vi "Get Case Structure (by Name).vi"(8 "error in (no error)":errorcluster, 10 "Case Structure name":string, 11 "VI ref in":refnum<vi>) -> (0 "error out":errorcluster, 1 "Found ?":bool, 2 "CaseStructure out":refnum<vi>, 3 "VI ref out":refnum<vi>)   [LabVIEW 2019, in "gRPC Template Creation Utility.lvlib"]
uses:
  gRPC Template Creation Utility.lvlib
  <vilib>/Utility/traverseref.llb/TRef TravTarget.ctl
  <vilib>/Utility/traverseref.llb/VI Scripting - Traverse.lvlib
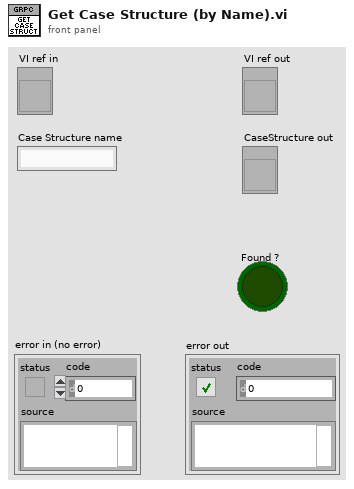
[diagram p1: front panel]
types:
  T1 = typedef "TRef TravTarget.ctl" = enum16{"FP", "BD", "Other"}
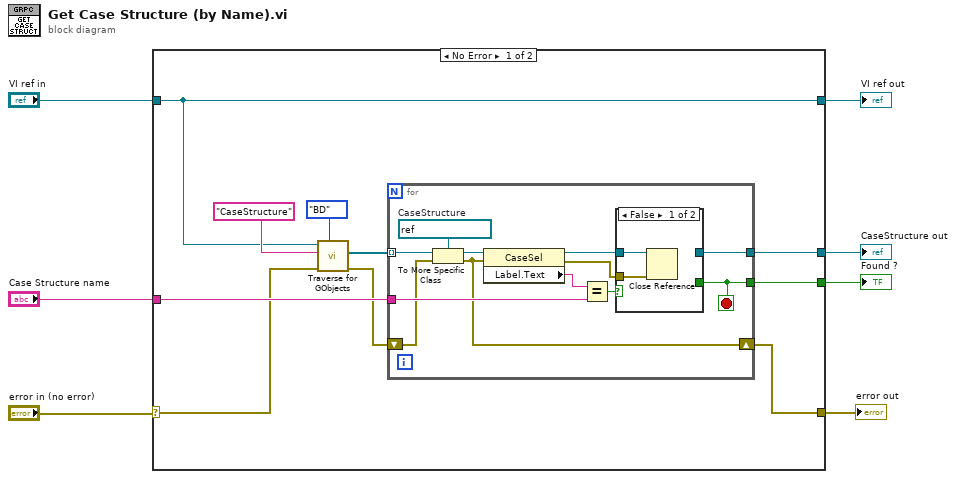
[diagram p0: block diagram]
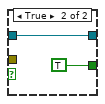
[diagram p2: hidden frame]
diagram:
  n1 = case shown="No Error" "error in (no error)" {
    selector: "error in (no error)" -> [w11 w35]
    tunnel: [w17 _] -> w7
    tunnel: "Case Structure name" -> [w16 _]
    tunnel: "VI ref in" -> [w8 w34]
    tunnel: [w12 _] -> w4
    tunnel: [w9 w35] -> w2
    tunnel: [w8 w34] -> w1
    frame No Error {
      n2 = call <vilib>:"Traverse for GObjects.vi"("Traverse Target"=TRef_TravTarget."BD", "error in (no error)"=w11, "Class Name"="CaseStructure", "VI Refnum"=w8) -> ("error out"=w10:errorcluster, "References"=w15:refnum<vi>[])  [unwired: 4 in, 2 out]
      n3 = for {
        tunnel: w15 -> [w27] mode=indexing
        tunnel: w16 -> [w25]
        tunnel: [w22] -> w17
        tunnel: [w18] -> w12
        shift-right: [w19] -> w9
        shift-left: w10 -> [w21]
        stop <- w18 stop-if-true
        w29 = refnum<vi> refnum  # CaseStructure
        n4 = To More Specific Class(target class=w29, reference=w27, error in=w21) -> (specific class reference=w28:refnum<vi>, error out=w19:errorcluster)
        n5 = property class="CaseSel"(reference=w28, error in=w19) -> (reference out=w23:refnum<vi>, error out=w20:errorcluster, "Label.Text"=w26:string)
        n6 = Equal?(x=w26, y=w25) -> (x = y?=w24:bool)
        n7 = case shown="False" w24 {
          tunnel: w23 -> [w31 w33]
          tunnel: [_ w33] -> w22
          tunnel: [_ TRUE] -> w18
          tunnel: w20 -> [w30 _]
          frame False {
            n8 = Close Reference(reference=w31, error in (no error)=w30) -> ()  [unwired: 1 out]
          }
          frame True {
          }
        }
      }
    }
    frame Error {
    }
  }
  "CaseStructure out" <- w7
  "VI ref out" <- w1
  "Found ?" <- w4
  "error out" <- w2
